vi "analyse.vi"(6 "cursors":T1, 8 "error in":errorcluster, 9 "Raw Data":waveform(dbl)[](graph)=[{"t0"=timestamp(0 s since 1904-01-01), "dt"=8.000000106811456e-10, "Y"=array[2502 elements]}, {"t0"=timestamp(0 s since 1904-01-01), "dt"=8.000000106811456e-10, "Y"=array[2502 elements]}], 10 "analysis_parameters":T2={"source"=enum."scope 1", "window"=enum."AB", "type"=enum."sum"}) -> (0 "error out":errorcluster, 2 "result":dbl)   [LabVIEW 2017, in "tools.lvlib"]
uses:
  tools.lvlib
  analysis_parameters.ctl
  cursors.ctl
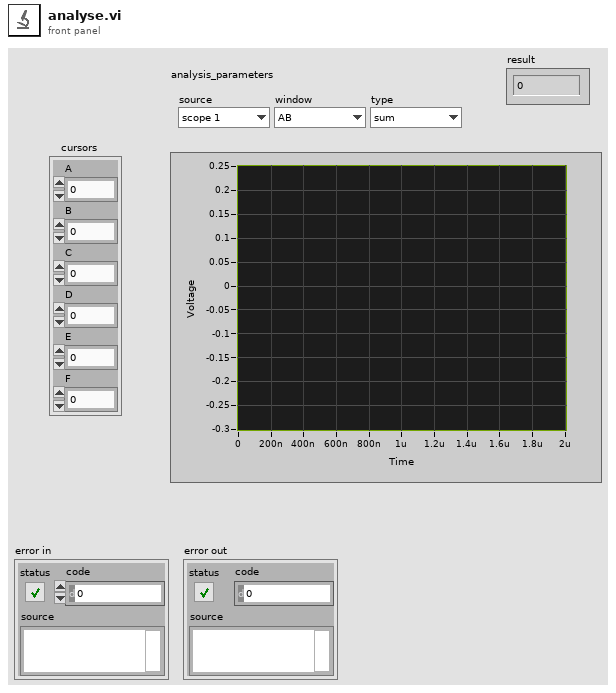
[diagram p1: front panel]
types:
  T1 = typedef "tools.lvlib/cursors.ctl" = cluster{"A":dbl, "B":dbl, "C":dbl, "D":dbl, "E":dbl, "F":dbl}
  T2 = typedef "tools.lvlib/analysis_parameters.ctl" = cluster{"source":enum16{"scope 0", "scope 1", "scope 2", "scope 3"}, "window":enum16{"AB", "CD", "EF"}, "type":enum16{"sum", "mean", "range"}}
  T3 = enum16{"scope 0", "scope 1", "scope 2", "scope 3"}
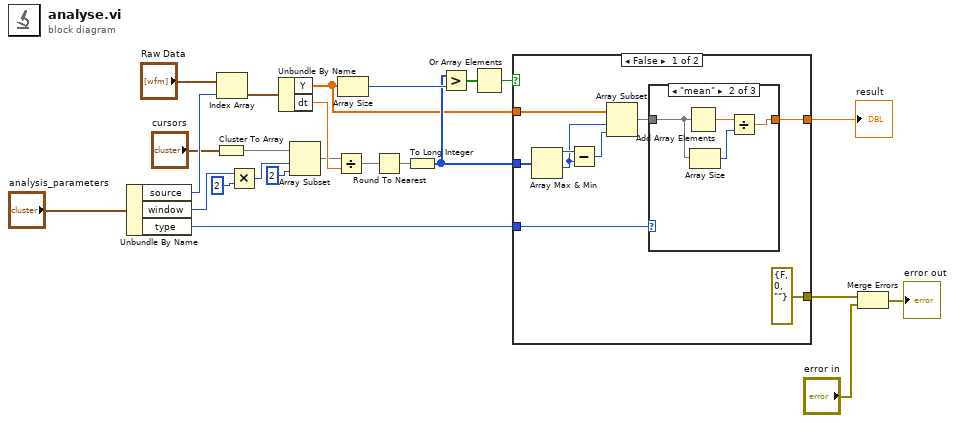
[diagram p0: block diagram]
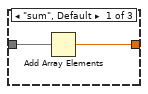
[diagram p2: hidden frame]
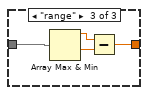
[diagram p3: hidden frame]
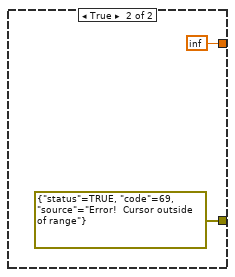
[diagram p4: hidden frame]
diagram:
  n1 = Unbundle By Name("analysis_parameters") -> ("source"=w22:T3, "window"=w21:enum16{"AB", "CD", "EF"}, "type"=w9:enum16{"sum", "mean", "range"})
  n2 = Cluster To Array(cluster="cursors") -> (array=w4:dbl[])
  n3 = Index Array(array="Raw Data", index=w22) -> (element=w7:waveform(dbl))
  n4 = Multiply(x=w21, y=2) -> (x*y=w15:i32)
  n5 = Unbundle By Name(w7) -> ("Y"=w6:dbl[], "dt"=w19:dbl)
  n6 = Array Subset(array=w4, index=w15, length=2 ("index")) -> (w13:dbl[])
  n7 = Divide(x=w13, y=w19) -> (x/y=w18:dbl[])
  n8 = Array Size(array=w6) -> (size(s)=w23:i32)
  n9 = Round To Nearest(number=w18) -> (nearest integer value=w17:dbl[])
  n10 = To Long Integer(number=w17) -> (32bit integer=w12:i32[])
  n11 = Greater?(x=w12, y=w23) -> (0:w11:bool[])
  n12 = Or Array Elements(Boolean array=w11) -> (logical OR=w16:bool)
  n13 = case shown="False" w16 {
    tunnel: w12 -> [w32 _]
    tunnel: w6 -> [w33 _]
    tunnel: w9 -> [w29 _]
    tunnel: [w28 inf] -> w8
    tunnel: [errorcluster {"status"=FALSE, "code"=0, "source"=""} ("error constant") errorcluster {"status"=TRUE, "code"=69, "source"="Error!  Cursor outside of range"} ("error constant")] -> w3
    frame False {
      n14 = Array Max & Min(array=w32) -> (max value=w31:i32, min value=w27:i32)  [unwired: 2 out]
      n15 = Subtract(x=w31, y=w27) -> (x-y=w30:i32)
      n16 = Array Subset(array=w33, index=w27, length=w30) -> (w26:dbl[])
      n17 = case shown="\"mean\"" w29 {
        tunnel: w26 -> [w35 w37 w43]
        tunnel: [w34 w38 w40] -> w28
        frame "sum", Default {
          n18 = Add Array Elements(numeric array=w35) -> (sum=w34:dbl)
        }
        frame "mean" {
          n19 = Add Array Elements(numeric array=w37) -> (sum=w39:dbl)
          n20 = Array Size(array=w37) -> (size(s)=w36:i32)
          n21 = Divide(x=w39, y=w36) -> (x/y=w38:dbl)
        }
        frame "range" {
          n22 = Array Max & Min(array=w43) -> (max value=w42:dbl, min value=w41:dbl)  [unwired: 2 out]
          n23 = Subtract(x=w42, y=w41) -> (x-y=w40:dbl)
        }
      }
    }
    frame True {
    }
  }
  "result" <- w8
  n24 = Merge Errors(w3, "error in") -> (→"error out":errorcluster)
